vi "StopGetPic.vi"() -> ()   [LabVIEW 2009]
panel:
  in  "Stop":bool
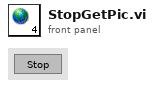
[diagram p1: front panel]
diagram:
